vi "Get Tx Generic Frame Header List.vi"(8 "error in":errorcluster, 11 "custom device ref in":T4 format="%.0x") -> (0 "error out":errorcluster, 2 "Frame Headers":T1[](array[typedef]) {"Frame header"."SequenceNumberOffset" items=["FDX_TX_FRAME_SEQ_OFFS_AUTO"=65535]; "Frame header"."SequenceNumberInit" items=["FDX_TX_FRAME_SEQ_INIT_AUTO"=65535, "FDX_TX_FRAME_SEQ_OFF"=65533]; "Frame header"."PhysErrorInjection" items=["FDX_TX_FRAME_ERR_OFF", "FDX_TX_FRAME_ERR_CRC", "FDX_TX_FRAME_ERR_ALI", "FDX_TX_FRAME_ERR_PRE", "FDX_TX_FRAME_ERR_PHY"]; "Frame header"."PayloadGenerationMode" items=["FDX_TX_FRAME_PGM_USER", "FDX_TX_FRAME_PGM_IP_PART", "FDX_TX_FRAME_PGM_IP_PART_TT", "FDX_TX_FRAME_PGM_IP_FULL", "FDX_TX_FRAME_PGM_IP_FULL_TT"]; "Frame header"."PayloadBufferMode" items=["FDX_TX_FRAME_PBM_STD", "FDX_TX_FRAME_PBM_MAC", "FDX_TX_FRAME_PBM_UDP", "FDX_TX_FRAME_PBM_FULL"]; "Frame header"."NetSelect" items=["FDX_TX_FRAME_DLY_A", "FDX_TX_FRAME_DLY_B", "FDX_TX_FRAME_BOTH", "FDX_TX_FRAME_ONLY_A", "FDX_TX_FRAME_ONLY_B"]; "Frame header"."FrameStartMode" items=["FDX_TX_FRAME_START_IFG", "FDX_TX_FRAME_START_PGWT", "FDX_TX_FRAME_START_TRG", "FDX_TX_FRAME_START_TRG_D"]}, 3 "custom device ref out":T4 format="%.0x")   [LabVIEW 2020, in "AIM ARINC 664 Scripting.lvlib"]
uses:
  <vilib>/NI VeriStand/Custom Device API/Custom Device Item Ref.ctl
  Shared/frame_tx_generic.ctl
  Shared/frame_tx_generic_seqNumberInit.ctl
  Shared/frame_tx_generic_seqNumberOffset.ctl
  Constants.vi
  AIM ARINC 664 Scripting.lvlib
  <vilib>/NI VeriStand/Custom Device API/Custom Device API.lvlib
  Import/AIM ARINC 664 Import.lvlib
  <vilib>/NI VeriStand/Custom Device API/Get Item Property (Variant).vi
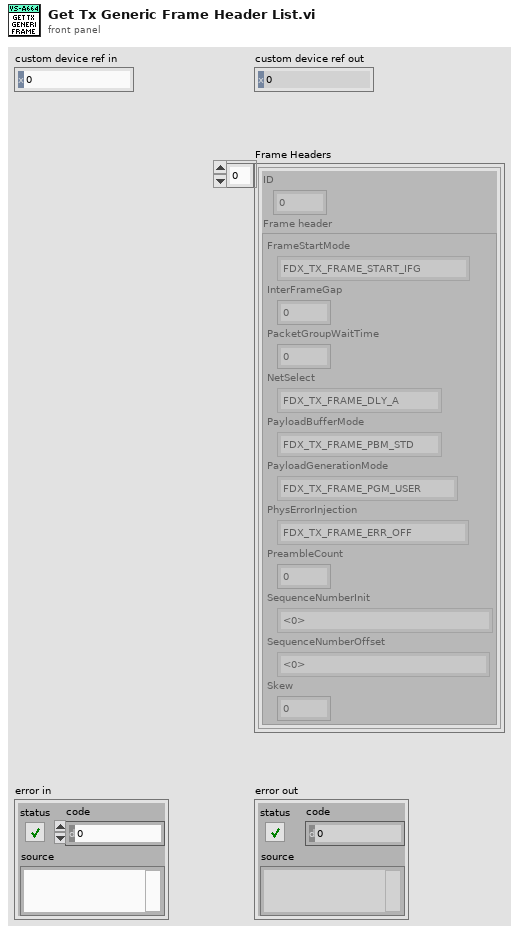
[diagram p1: front panel]
types:
  T1 = typedef "AIM ARINC 664 Import.lvlib/frame_tx_generic.ctl" = cluster{"ID":i32, "Frame header":cluster{"FrameStartMode":i32, "InterFrameGap":i32, "PacketGroupWaitTime":i32, "NetSelect":i32, "PayloadBufferMode":i32, "PayloadGenerationMode":i32, "PhysErrorInjection":i32, "PreambleCount":i32, "SequenceNumberInit":T2, "SequenceNumberOffset":T3, "Skew":i32}}
  T2 = typedef "AIM ARINC 664 Import.lvlib/frame_tx_generic_seqNumberInit.ctl" = i32
  T3 = typedef "AIM ARINC 664 Import.lvlib/frame_tx_generic_seqNumberOffset.ctl" = i32
  T4 = typedef "Custom Device API.lvlib/Custom Device Item Ref.ctl" = u64
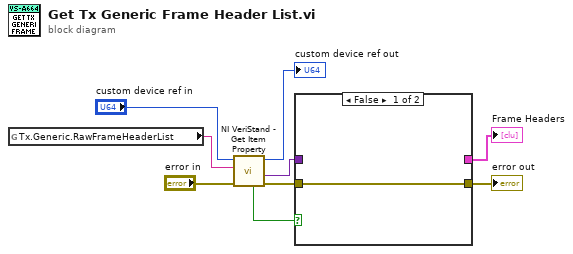
[diagram p0: block diagram]
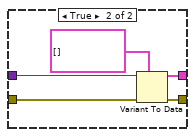
[diagram p2: hidden frame]
diagram:
  n1 = global read "Constants.vi" "Tx.Generic.RawFrameHeaderList"() -> (w6:string)
  n2 = call-poly <vilib>:"NI VeriStand - Get Item Property.vi"("error in (no error)"="error in", "Property Name"=w6, "Item Ref in"="custom device ref in") -> ("error out"=w5:errorcluster, "Value"=w3:variant, "Item Ref out"=→"custom device ref out":T4, "Found?"=w4:bool)  [unwired: 5 in]
  n3 = case shown="False" w4 {
    tunnel: w5 -> [w10 w15]
    tunnel: w3 -> [_ w14]
    tunnel: [_ w12] -> w1
    tunnel: [w10 w11] -> w2
    frame False {
    }
    frame True {
      n4 = Variant To Data(error in=w15, type=T1[] [] ("Frame Headers"), Variant=w14) -> (data=w12:T1[], error out=w11:errorcluster)
    }
  }
  "error out" <- w2
  "Frame Headers" <- w1
